vi "Global - Parameters.vi"() -> ()   [LabVIEW 2018]
panel:
  in  "PV":dbl
  # "Propotional Valve"
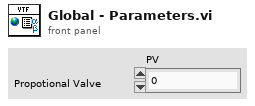
[diagram p1: front panel]
diagram:
